vi "Actor Core.vi"(8 "Error In":errorcluster, 11 "Test LNA in":refnum<class "TestLNA.lvclass">) -> (0 "Error Out":errorcluster, 3 "Actor out":refnum<class "Actor.lvclass">)   [LabVIEW 2015, in "TestLNA.lvlib" / "TestLNA.lvclass"]
doc: "(<B>Filename</B>: Actor Framework.lvlib:Actor.lvclass:Actor Core.vi)\n\nReceives messages to the actor, reacts to them, and initiates any error handling that may shut the actor down.\n\nDescendant classes may override this VI to append parallel tasks for the actor to complete while it handles messages. Overrides use the Call Parent Method node."
uses:
  TestLNA.lvclass
  <vilib>/ActorFramework/Actor/Actor.lvclass
  <vilib>/NI/Actors/Linked Network Actor/Linked Network Actor/Linked Network Actor.lvclass
  LNA Messages/LNA Connection Status Msg/LNA Connection Status Msg.lvclass
  LNA Messages/LNA Return Message Msg/LNA Return Message Msg.lvclass
  CSPP_Core/Actors/CS++BaseActor/CS++BaseActor.lvclass/CS++BaseActor.ctl
  TestLNA.lvclass/TestLNA.ctl
  <vilib>/NI/Actors/Linked Network Actor/Linked Network Actor/Linked Network Actor.lvclass/Linked Network Actor.ctl
  CSPP_Core/Actors/CS++BaseActor/CS++BaseActor.lvclass
  <vilib>/NI/Actors/Linked Network Actor/Linked Network Actor Messages/Connect Msg/Connect Msg.lvclass
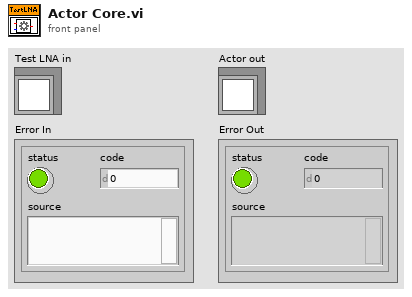
[diagram p1: front panel]
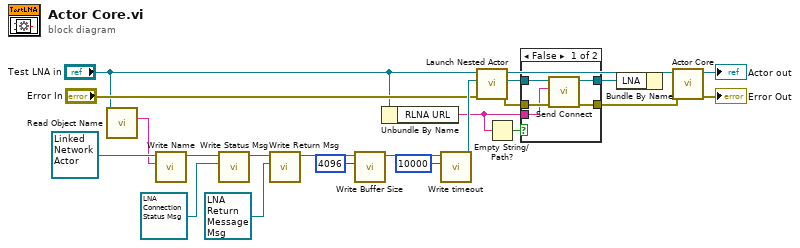
[diagram p0: block diagram]
diagram:
  n1 = call "Read Object Name.vi"("CS++BaseActor in"="Test LNA in") -> ("Object Name"=w1:string)  [unwired: 8 in, 2 out]
  n2 = call <vilib>:"Write Name.vi"("Name"=w1, "Network Actor in"=refnum<class "Linked Network Actor.lvclass"> refnum ("Linked Network Actor.lvlib:Linked Network Actor.lvclass")) -> ("Network Actor out"=w14:refnum<class "Linked Network Actor.lvclass">)  [unwired: 9 in]
  n3 = call <vilib>:"Write Status Msg.vi"("Status Msg"=refnum<class "LNA Connection Status Msg.lvclass"> refnum ("Test LNA.lvlib:LNA Connection Status Msg.lvclass"), "Network Actor in"=w14) -> ("Network Actor out"=w15:refnum<class "Linked Network Actor.lvclass">)  [unwired: 9 in]
  n4 = call <vilib>:"Write Return Msg.vi"("Return Msg"=refnum<class "LNA Return Message Msg.lvclass"> refnum ("Test LNA.lvlib:LNA Return Message Msg.lvclass"), "Linked Network Actor in"=w15) -> ("Linked Network Actor out"=w13:refnum<class "Linked Network Actor.lvclass">)  [unwired: 9 in]
  n5 = call <vilib>:"Write Buffer Size.vi"("Buffer Size"=4096, "Network Actor in"=w13) -> ("Network Actor out"=w20:refnum<class "Linked Network Actor.lvclass">)  [unwired: 9 in]
  n6 = Unbundle By Name("Test LNA in") -> ("RLNA URL"=w2:string)
  n7 = call <vilib>:"Write timeout.vi"("timeout"=10000, "Network Actor in"=w20) -> ("Network Actor out"=w17:refnum<class "Linked Network Actor.lvclass">)  [unwired: 9 in]
  n8 = call <vilib>:"Launch Nested Actor.vi"("error in (no error)"="Error In", "Nested Actor"=w17, "Caller Actor in"="Test LNA in") -> ("error out"=w7:errorcluster, "Nested Actor's Enqueuer"=w8:refnum<class "Message Enqueuer.lvclass">, "Caller Actor out"=w10:refnum<class "TestLNA.lvclass">)  [unwired: 6 in]
  n9 = Empty String/Path?(string/path=w2) -> (empty?=w3:bool)
  n10 = case shown="False" w3 {
    tunnel: w8 -> [w28 w30]
    tunnel: w7 -> [w27 w29]
    tunnel: [w26 w29] -> w6
    tunnel: [w25 w30] -> w5
    tunnel: w2 -> [w24 _]
    frame False {
      n11 = call <vilib>:"Send Connect.vi"("error in (no error)"=w27, "URL"=w24, "Message Enqueuer"=w28) -> ("error out"=w26:errorcluster, "Message Enqueuer out"=w25:refnum<class "Message Enqueuer.lvclass">)  [unwired: 7 in]
    }
    frame True {
    }
  }
  n12 = Bundle By Name(cluster=w10, "LNA"=w5) -> (w9:refnum<class "TestLNA.lvclass">)
  n13 = call-parent "Actor Core.vi"("error in"=w6, "CS++BaseActor in"=w9) -> ("error out"=→"Error Out":errorcluster, "Actor out"=→"Actor out":refnum<class "Actor.lvclass">)  [unwired: 8 in]
